vi "MoveZmicroSwitch1.vi"(0 "Z":dbl=60.0, 1 "Zspeed":dbl=25.0, 2 "controller in":refnum<k24>, 3 "error in (no error)":errorcluster) -> (7 "MoveZ":string, 8 "controller out":refnum<k24>, 9 "data":bool[](array[boolean]), 10 "error out":errorcluster)   [LabVIEW 2021]
uses:
  C:/Users/TTUHEP/Documents/LabVIEW/Other Models/2010/Bin/Aerotech.A3200.dll
  Other Models/2010/Bin/Aerotech.A3200.dll
  Other Models/2010/Motion/AbortSingle.vi
panel:
  # "Move along Z, abs coordinates, with speed v mm/s"
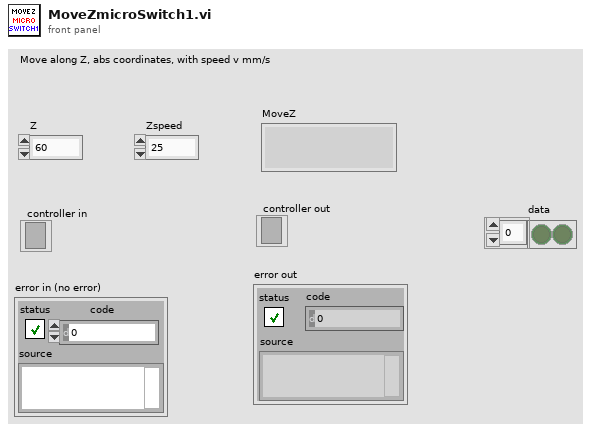
[diagram p1: front panel]
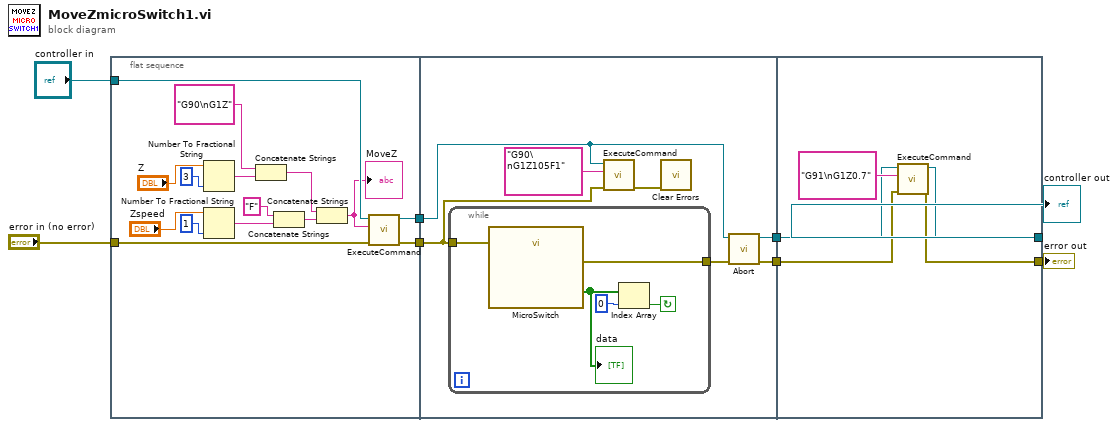
[diagram p0: block diagram]
diagram:
  n1 = flat-sequence {
    tunnel: "error in (no error)" -> [w23]
    tunnel: "controller in" -> [w22]
    tunnel: [w21] -> w8
    tunnel: [w20] -> w7
    tunnel: w8 -> [w27]
    tunnel: w7 -> [w26]
    tunnel: [w24] -> w2
    tunnel: [w25] -> w1
    tunnel: [w38] -> w6
    tunnel: [w36] -> w3
    tunnel: w2 -> [w37]
    tunnel: w1 -> [w39]
    frame #0 {
      n2 = Number To Fractional String(number="Z", precision (6)=i16 3) -> (F-format string=w15:string)  [unwired: 2 in]
      n3 = Number To Fractional String(number="Zspeed", precision (6)=i16 1) -> (F-format string=w18:string)  [unwired: 2 in]
      n4 = Concatenate Strings("G90\nG1Z", w15) -> (w16:string)
      n5 = Concatenate Strings("F" ("string"), w18) -> (w19:string)
      n6 = Concatenate Strings(w16, w19) -> (w9:string)
      "MoveZ" <- w9
      n7 = call "ExecuteCommand.vi"("error in (no error)"=w23, "Command Code"=w9, "controller in"=w22) -> ("error out"=w20:errorcluster, "controller out"=w21:refnum<k24>)  [unwired: 6 in, 1 out]
    }
    frame #1 {
      n8 = while {
        tunnel: [w35] -> w29
        tunnel: w26 -> [w34]
        stop <- w32 continue-if-true
        n9 = call "MicroSwitch"("error in"=w34) -> ("data"=w33:bool[], "error out"=w35:errorcluster)  [unwired: 16 in, 1 out]
        "data" <- w33
        n10 = Index Array(array=w33, index=0) -> (element=w32:bool)
      }
      n11 = call "ExecuteCommand.vi"("error in (no error)"=w26, "Command Code"="G90\nG1Z105F1", "controller in"=w27) -> ("error out"=w28:errorcluster)  [unwired: 6 in, 2 out]
      n12 = call <vilib>:"Clear Errors.vi"("error in (no error)"=w28) -> ()  [unwired: 5 in, 2 out]
      n13 = call-poly "Abort.vi"("error in (no error)"=w29, "controller in"=w27) -> ("error out"=w24:errorcluster, "controller out"=w25:refnum<k24>)  [unwired: 8 in]
    }
    frame #2 {
      n14 = call "ExecuteCommand.vi"("error in (no error)"=w37, "Command Code"="G91\nG1Z0.7", "controller in"=w39) -> ("error out"=w36:errorcluster, "controller out"=w38:refnum<k24>)  [unwired: 6 in, 1 out]
    }
  }
  "controller out" <- w6
  "error out" <- w3
